vi "excel.vi"() -> ()   [LabVIEW 2020]
uses:
  <vilib>/Utility/NIReport.llb/Excel/NI_Excel.lvclass
  <vilib>/addons/_office/NI_ReportGenerationToolkit.lvlib
  <vilib>/Utility/NIReport.llb/NI_report.lvclass
  <vilib>/addons/_office/excel.llb/Excel Get Data ([dbl]).vi
panel:
  out "Array 2":dbl[][](array[numeric])
  out "Array":dbl[](array[numeric])
  out "Sheet 1 Data":dbl[][](array[numeric]) format="%.2f"
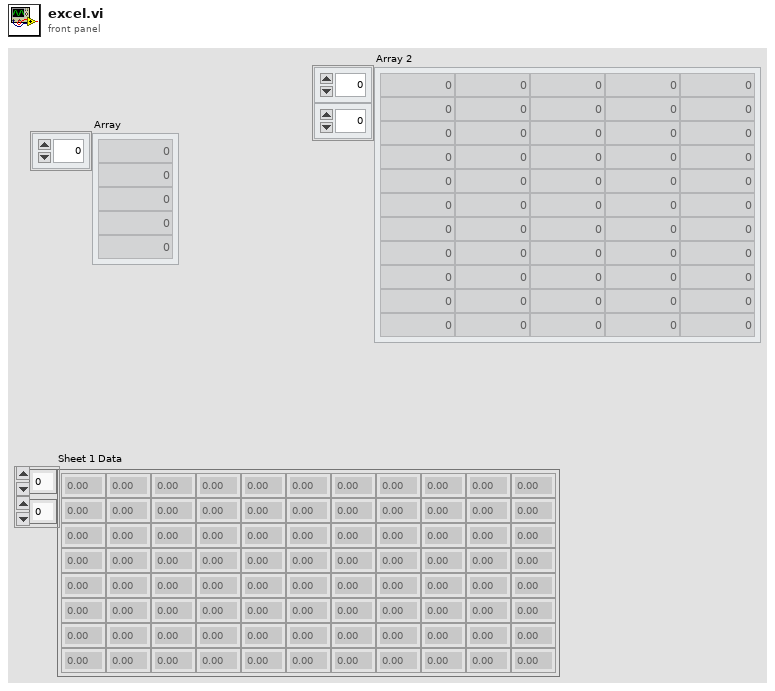
[diagram p1: front panel]
types:
  T1 = enum16{"Standard Report", "HTML", "Word", "Excel"}
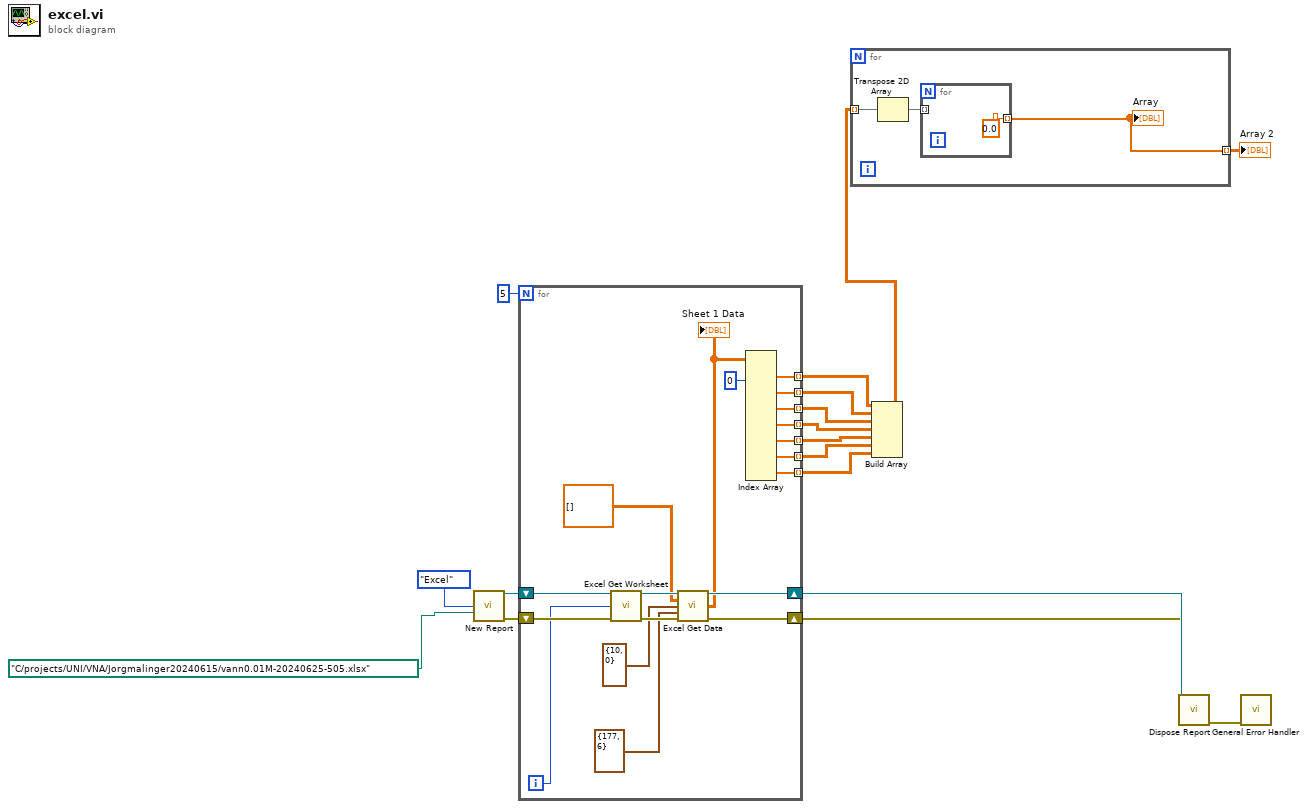
[diagram p0: block diagram]
diagram:
  n1 = call <vilib>:"New Report.vi"("report type"=T1."Excel", "template (empty)"=path "C:/projects/UNI/VNA/Jorgmalinger20240615/vann0.01M-20240625-505.xlsx" ("file path (dialog if empty)")) -> ("report out"=w17:refnum<class "NI_report.lvclass">, "error out"=w14:errorcluster)  [unwired: 4 in, 8 out]
  n2 = for {
    N: 5 -> [_]
    shift-right: [w33] -> w15
    shift-left: w17 -> [w36]
    shift-right: [w29] -> w12
    shift-left: w14 -> [w32]
    tunnel: [w26] -> w8 mode=indexing
    tunnel: [w23] -> w7 mode=indexing
    tunnel: [w22] -> w5 mode=indexing
    tunnel: [w21] -> w4 mode=indexing
    tunnel: [w20] -> w3 mode=indexing
    tunnel: [w19] -> w2 mode=indexing
    tunnel: [w18] -> w1 mode=indexing
    i -> [w27]
    n3 = call <vilib>:"Excel Get Worksheet.vi"("report in"=w36, "worksheet index (0)"=w27, "error in (no error)"=w32) -> ("report out"=w35:refnum<class "NI_report.lvclass">, "error out"=w31:errorcluster)  [unwired: 11 out]
    n4 = call-poly <vilib>:"Excel Get Data.vi"("report in"=w35, "data type"=dbl[][] [], "start (-1, -1)"=cluster{"row":i32, "column":i32} {"row"=10, "column"=0}, "end (-1, -1)"=cluster{"row":i32, "column":i32} {"row"=177, "column"=6}, "error in (no error)"=w31) -> ("report out"=w33:refnum<class "NI_report.lvclass">, "data"=w24:dbl[][], "error out"=w29:errorcluster)  [unwired: 8 out]
    "Sheet 1 Data" <- w24
    n5 = Index Array(array=w24, index (col) #1=0 ("disabled index (col)")) -> (element #1=w26:dbl[], element #2=w23:dbl[], element #3=w22:dbl[], element #4=w21:dbl[], element #5=w20:dbl[], element #6=w19:dbl[], element #7=w18:dbl[])  [unwired: 13 in]
  }
  n6 = Build Array(w8, w7, w5, w4, w3, w2, w1) -> (w6:dbl[][][])
  n7 = for {
    tunnel: w6 -> [w37] mode=indexing
    tunnel: [w38] -> w9 mode=indexing
    n8 = Transpose 2D Array(2D array=w37) -> (transposed array=w39:dbl[][])
    n9 = for {
      tunnel: w39 -> [_] mode=indexing
      tunnel: [0.0 ("Numeric")] -> w38 mode=indexing
    }
    "Array" <- w38
  }
  "Array 2" <- w9
  n10 = call-dynamic "Dispose Report.vi"("report in"=w15, "error in (no error)"=w12) -> ("error out"=w13:errorcluster)  [unwired: 3 in, 10 out]
  n11 = call <vilib>:"General Error Handler.vi"("error in (no error)"=w13) -> ()  [unwired: 3 in, 12 out]
